vi "Add Tx Generic Section and Status Channels.vi"(8 "error in":errorcluster, 10 "Tx generic configuration":T1={"tx_generic_setup"={"QueueSizeIn"=0, "Count"=12, "StartMode"=1}, "Frame Headers"=[]} {"Frame Headers"."Parameters"."Parameter"."encoding" items=["BNR", "BCD", "Discrete"]; "Frame Headers"."Frame header"."SequenceNumberOffset" items=["FDX_TX_FRAME_SEQ_OFFS_AUTO"=65535]; "Frame Headers"."Frame header"."SequenceNumberInit" items=["FDX_TX_FRAME_SEQ_INIT_AUTO"=65535, "FDX_TX_FRAME_SEQ_OFF"=65533]; "Frame Headers"."Frame header"."PhysErrorInjection" items=["FDX_TX_FRAME_ERR_OFF", "FDX_TX_FRAME_ERR_CRC", "FDX_TX_FRAME_ERR_ALI", "FDX_TX_FRAME_ERR_PRE", "FDX_TX_FRAME_ERR_PHY"]; "Frame Headers"."Frame header"."PayloadGenerationMode" items=["FDX_TX_FRAME_PGM_USER", "FDX_TX_FRAME_PGM_IP_PART", "FDX_TX_FRAME_PGM_IP_PART_TT", "FDX_TX_FRAME_PGM_IP_FULL", "FDX_TX_FRAME_PGM_IP_FULL_TT"]; "Frame Headers"."Frame header"."PayloadBufferMode" items=["FDX_TX_FRAME_PBM_STD", "FDX_TX_FRAME_PBM_MAC", "FDX_TX_FRAME_PBM_UDP", "FDX_TX_FRAME_PBM_FULL"]; "Frame Headers"."Frame header"."NetSelect" items=["FDX_TX_FRAME_DLY_A"=0, "FDX_TX_FRAME_DLY_B"=1, "FDX_TX_FRAME_BOTH "=3, "FDX_TX_FRAME_ONLY_A"=4, "FDX_TX_FRAME_ONLY_B "=5]; "Frame Headers"."Frame header"."FrameStartMode" items=["FDX_TX_FRAME_START_IFG", "FDX_TX_FRAME_START_PGWT", "FDX_TX_FRAME_START_TRG", "FDX_TX_FRAME_START_TRG_D"]; "tx_generic_setup"."StartMode" items=["FDX_STOP", "FDX_START", "FDX_START_TRG", "FDX_START_TIME"]}, 11 "port ref":T9 format="%.0x") -> (0 "error out":errorcluster, 3 "port ref out":T9 format="%.0x")   [LabVIEW 2020, in "AIM ARINC 664 Scripting.lvlib"]
doc: "Add a Tx Generic pages based on the configuration input."
uses:
  AIM ARINC 664 Scripting.lvlib
  <vilib>/NI VeriStand/Custom Device API/Custom Device Item Ref.ctl
  Import/_typedefs/session_tx_generic.ctl
  Import/_typedefs/tx_generic_setup.ctl
  Import/_typedefs/frame_tx_generic.ctl
  Import/_typedefs/frame_tx_generic_seqNumberInit.ctl
  Import/_typedefs/frame_tx_generic_seqNumberOffset.ctl
  Import/_typedefs/frame_parameter.ctl
  Import/_typedefs/frame_parameter_definition.ctl
  Shared/Encoding (Arinc664).ctl
  <vilib>/Utility/SystemLogging/NI_SystemLogging.lvlib
  Import/AIM ARINC 664 Import.lvlib
  <vilib>/NI VeriStand/Custom Device API/Custom Device API.lvlib
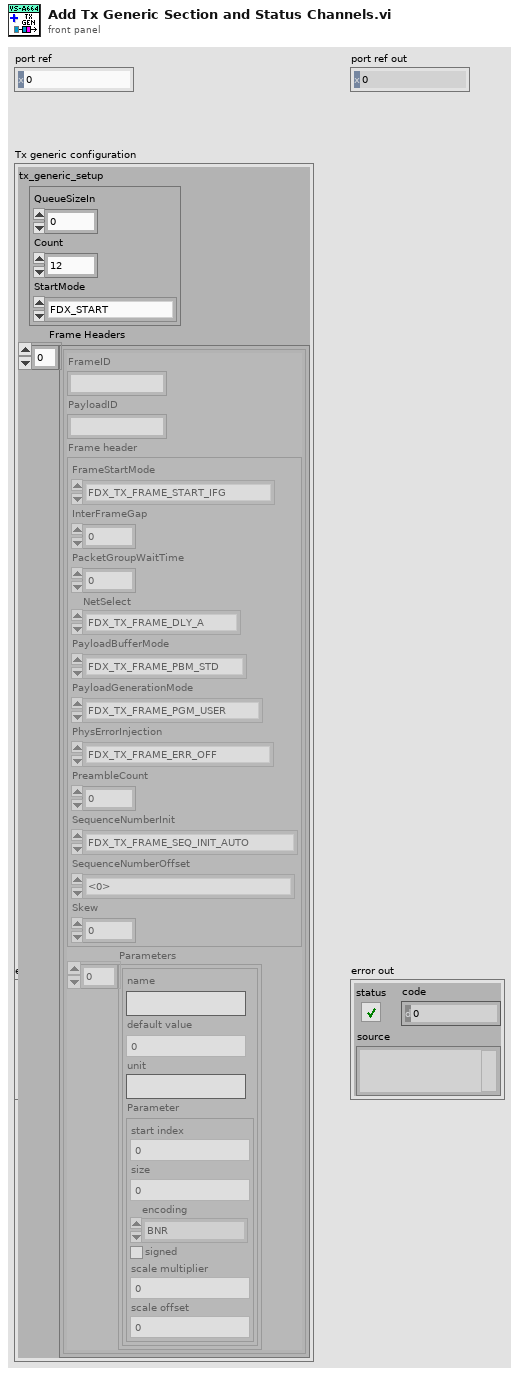
[diagram p1: front panel]
types:
  T1 = typedef "AIM ARINC 664 Import.lvlib/session_tx_generic.ctl" = cluster{"tx_generic_setup":T2, "Frame Headers":T3[]}
  T2 = typedef "AIM ARINC 664 Import.lvlib/tx_generic_setup.ctl" = cluster{"QueueSizeIn":u32, "Count":i32, "StartMode":i32}
  T3 = typedef "AIM ARINC 664 Import.lvlib/frame_tx_generic.ctl" = cluster{"FrameID":string, "PayloadID":string, "Frame header":cluster{"FrameStartMode":i32, "InterFrameGap":i32, "PacketGroupWaitTime":i32, "NetSelect":u32, "PayloadBufferMode":i32, "PayloadGenerationMode":i32, "PhysErrorInjection":i32, "PreambleCount":i32, "SequenceNumberInit":T4, "SequenceNumberOffset":T5, "Skew":i32}, "Parameters":T6[]}
  T4 = typedef "AIM ARINC 664 Import.lvlib/frame_tx_generic_seqNumberInit.ctl" = i32
  T5 = typedef "AIM ARINC 664 Import.lvlib/frame_tx_generic_seqNumberOffset.ctl" = i32
  T6 = typedef "AIM ARINC 664 Import.lvlib/frame_parameter.ctl" = cluster{"name":string, "default value":dbl, "unit":string, "Parameter":T7}
  T7 = typedef "AIM ARINC 664 Import.lvlib/frame_parameter_definition.ctl" = cluster{"start index":i32, "size":i32, "encoding":T8, "signed":bool, "scale multiplier":dbl, "scale offset":dbl}
  T8 = typedef "Encoding (Arinc664).ctl" = u16
  T9 = typedef "Custom Device API.lvlib/Custom Device Item Ref.ctl" = u64
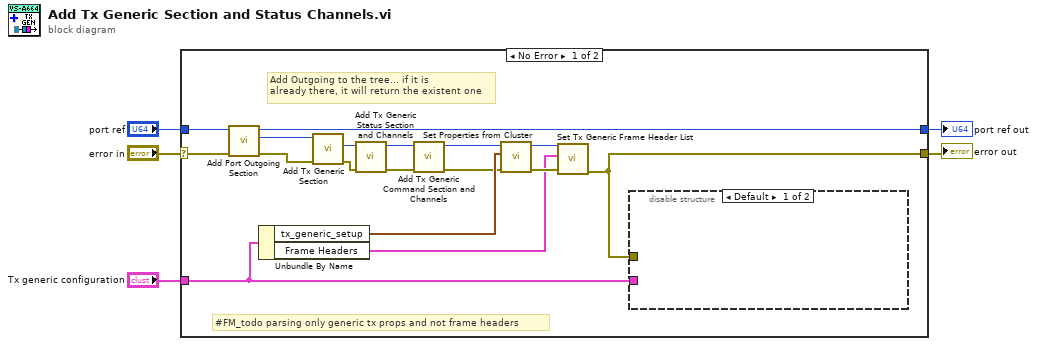
[diagram p0: block diagram]
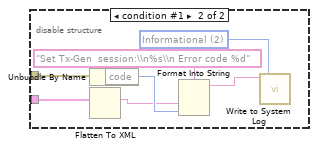
[diagram p2: hidden frame]
diagram:
  n1 = case shown="No Error" "error in" {
    selector: "error in" -> [w16 w31]
    tunnel: "port ref" -> [w22 w30]
    tunnel: "Tx generic configuration" -> [w15 _]
    tunnel: [w11 w31] -> w3
    tunnel: [w21 w30] -> w2
    frame No Error {
      # "#FM_todo parsing only generic tx props and not frame headers"
      # "Add Outgoing to the tree... if it is \nalready there, it will return the existent one"
      n2 = call "Add Port Outgoing Section.vi"("error in"=w16, "ports ref"=w22) -> ("error out"=w18:errorcluster, "port outgoing ref out"=w20:T9, "ports ref out"=w21:T9)  [unwired: 7 in]
      n3 = Unbundle By Name(w15) -> ("tx_generic_setup"=w14:T2, "Frame Headers"=w10:T3[])
      n4 = call "Add Tx Generic Section.vi"("error in"=w18, "port outgoing ref"=w20) -> ("error out"=w19:errorcluster, "Tx generic section ref out"=w17:T9)  [unwired: 7 in, 1 out]
      n5 = call "Add Tx Generic Status Section and Channels.vi"("error in"=w19, "Tx generic ref in"=w17) -> ("error out"=w8:errorcluster, "Tx generic ref out"=w9:T9)  [unwired: 6 in, 2 out]
      n6 = call "Add Tx Generic Command Section and Channels.vi"("error in"=w8, "Tx generic ref in"=w9) -> ("error out"=w7:errorcluster, "Tx generic ref out"=w6:T9)  [unwired: 6 in, 2 out]
      n7 = call "Set Properties from Cluster.vi"("error in"=w7, "Variant Cluster"=w14, "item ref in"=w6) -> ("error out"=w13:errorcluster, "item ref out"=w12:T9)  [unwired: 7 in]
      n8 = call "Set Tx Generic Frame Header List.vi"("error in"=w13, "Frame Headers"=w10, "custom device ref in"=w12) -> ("error out"=w11:errorcluster)  [unwired: 7 in, 1 out]
      n9 = disable-structure shown="Default" {
        disable-tunnel: w11 -> [_ w25]
        disable-tunnel: w15 -> [_ w24]
        frame condition #0 (active) {
        }
        frame condition #1 {
          w27 = 2 items=["Error", "Warning", "Informational"] ("severity")
          n10 = Unbundle By Name(w25) -> ("code"=w26:i32)
          n11 = Flatten To XML(6:w24) -> (2:w23:string)
          n12 = Format Into String(format string="Set Tx-Gen  session:\\n%s\\n Error code %d", w23, w26) -> (resulting string=w28:string)  [unwired: 2 in, 1 out]
          n13 = call <vilib>:"Write to System Log.vi"("severity"=w27, "message"=w28) -> ()  [unwired: 9 in, 1 out]
        }
      }
    }
    frame Error {
    }
  }
  "port ref out" <- w2
  "error out" <- w3
